vi "setInputParameter.vi"(8 "error in (no error)":errorcluster, 10 "input":variant, 11 "HGF_Visitable.lvclass in":refnum<class "HGF_Visitable.lvclass">) -> (0 "error out":errorcluster, 3 "HGF_Visitable.lvclass out":refnum<class "HGF_Visitable.lvclass">)   [LabVIEW 2014, in "HGF_BaseClasses.lvlib" / "HGF_Visitable.lvclass"]
doc: "Set input parameter attribute."
uses:
  HGF_Visitable.lvclass
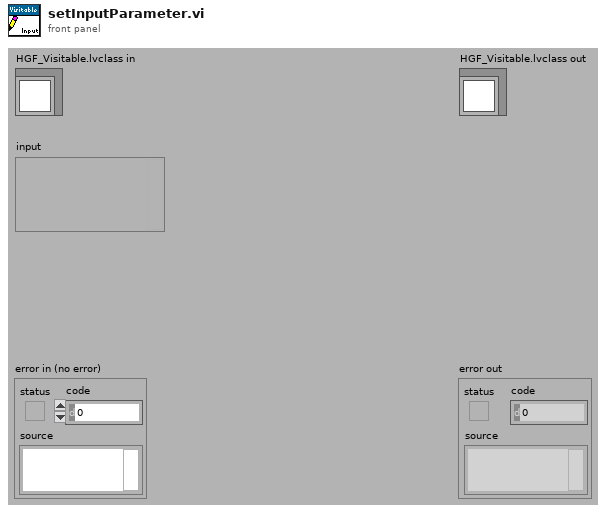
[diagram p1: front panel]
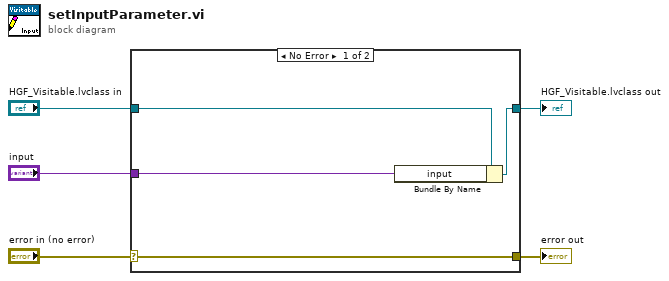
[diagram p0: block diagram]
diagram:
  n1 = case shown="No Error" "error in (no error)" {
    selector: "error in (no error)" -> [w9 w10]
    tunnel: [w9 w10] -> w4
    tunnel: [w7 w11] -> w2
    tunnel: "HGF_Visitable.lvclass in" -> [w8 w11]
    tunnel: "input" -> [w6 _]
    frame No Error {
      n2 = Bundle By Name(cluster=w8, "input"=w6) -> (w7:refnum<class "HGF_Visitable.lvclass">)
    }
    frame Error {
    }
  }
  "error out" <- w4
  "HGF_Visitable.lvclass out" <- w2
